vi "IMAQdx Wait for IO Signal Edge.vi"(6 "Signal Edge":u32(ring) items=["Rising Edge", "Falling Edge"], 7 "Timeout (ms)":i32=5000, 8 "error in":errorcluster, 9 "Signal Number":u32, 10 "Signal Type":u32(ring) items=["TTL", "RTSI", "Iso In", "Iso Out"], 11 "Session In":T1) -> (0 "error out":errorcluster, 3 "Session Out":T1)   [LabVIEW 2020, in "NI_Vision_Acquisition_Software.lvlib"]
doc: "Synchronous wait for an edge on an IO signal."
uses:
  NI_Vision_Acquisition_Software.lvlib
  IMAQdx.ctl
  niimaqdx.dll
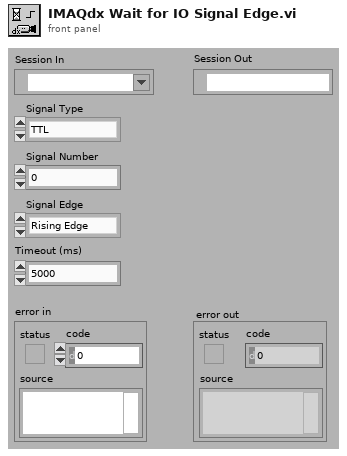
[diagram p1: front panel]
types:
  T1 = typedef "IMAQdx.ctl" = refnum<k21>
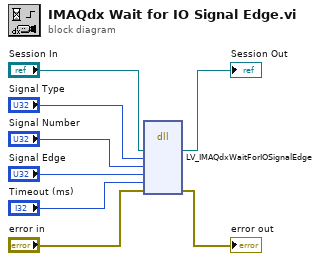
[diagram p0: block diagram]
diagram:
  n1 = dll-call lib="niimaqdx.dll" fn="LV_IMAQdxWaitForIOSignalEdge"("refnum"="Session In", "signalType"="Signal Type", "signalNumber"="Signal Number", "signalEdge"="Signal Edge", "timeoutMs"="Timeout (ms)", "error"="error in") -> ("refnum"=→"Session Out":T1, "error"=→"error out":errorcluster)  [unwired: 8 in, 2 out]
